vi "Read Current.vi"(0 "reference in":refnum<class "Power Supply.lvclass">, 5 "error in (no error)":errorcluster) -> (14 "reference out":refnum<class "Power Supply.lvclass">, 18 "Power Supply Current Reading":dbl format="%.4f", 19 "error out":errorcluster)   [LabVIEW 2017, in "Power Supply.lvclass"]
uses:
  Power Supply.lvclass
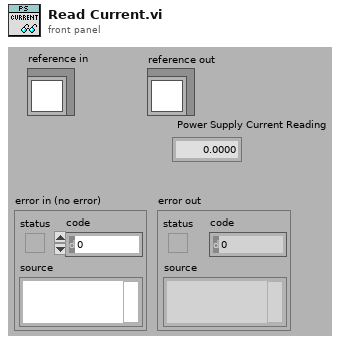
[diagram p1: front panel]
types:
  T1 = typedef "Power Supply.lvclass/ObjectAttributes.ctl" = cluster{"Power Supply Chain VISA Session":refnum<visa-resource-name>, "Power Supply Chain Address":i16, "Power Supply Open/Close Status":bool, "Power Supply Voltage Setting":dbl, "Power Supply Current Setting":dbl, "Power Supply Voltage Reading":dbl, "Power Supply Current Reading":dbl, "Power Supply Status":T2, "Power Supply Error":T3, "Fault Register":u8, "Power Supply Error":bool}
  T2 = typedef "Power Supply.lvclass/Power Supply Status.ctl" = enum16{"Closed", "Open"}
  T3 = typedef "Power Supply.lvclass/Power Supply Error.ctl" = enum16{"None", "Read Error"}
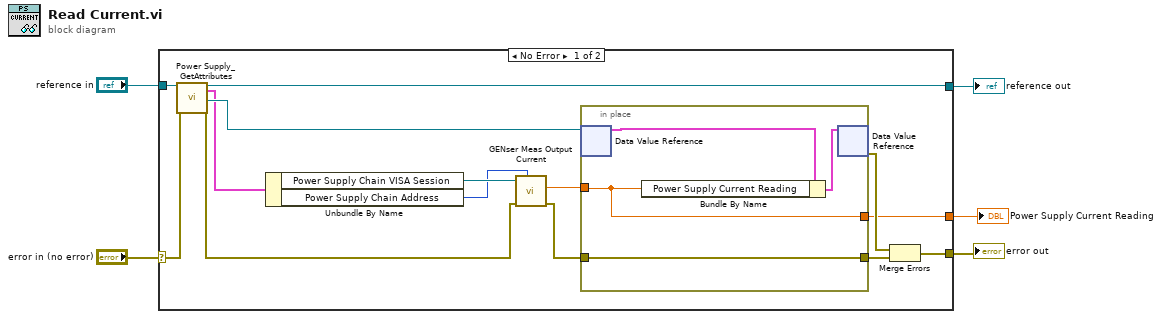
[diagram p0: block diagram]
diagram:
  n1 = case shown="No Error" "error in (no error)" {
    selector: "error in (no error)" -> [w18 w25]
    tunnel: [w15 w25] -> w4
    tunnel: [w16 w24] -> w2
    tunnel: "reference in" -> [w19 w24]
    tunnel: [w12 _] -> w1
    frame No Error {
      n2 = call "Power Supply_GetAttributes.vi"("reference in"=w19, "error in (no error)"=w18) -> ("reference out"=w16:refnum<class "Power Supply.lvclass">, "Data"=w9:T1, "DataRef"=w14:refnum<data-value>, "error out"=w7:errorcluster)  [unwired: 14 in]
      n3 = Unbundle By Name(w9) -> ("Power Supply Chain VISA Session"=w11:refnum<visa-resource-name>, "Power Supply Chain Address"=w10:i16)
      n4 = call <instrlib>:"GENser Meas Output Current.vi"("GEN Addr"=w10, "error"=w7, "VISA"=w11) -> ("error out"=w6:errorcluster, "Output Current"=w8:dbl)  [unwired: 6 in, 1 out]
      n5 = in-place {
        in-place-border: w6 -> [w20]
        in-place-border: [w20] -> w13
        in-place-border: [w21] -> w12
        in-place-border: w8 -> [w21]
        n6 = in-place-dvr #1(w14) -> (w22:T1)  [unwired: 1 out]
        n7 = Bundle By Name(cluster=w22, "Power Supply Current Reading"=w21) -> (w23:T1)
        n8 = in-place-dvr #1(w23) -> (w17:errorcluster)  [unwired: 1 out]
      }
      n9 = Merge Errors(w17, w13) -> (w15:errorcluster)
    }
    frame Error {
    }
  }
  "error out" <- w4
  "reference out" <- w2
  "Power Supply Current Reading" <- w1
